vi "WriteLog.vi"(7 "subsystem":string, 8 "data":dbl, 9 "tag":string, 10 "log level":T2(ring)=enum."default", 11 "logger":T1) -> (2 "error code":i32 format="%0.0f", 3 "logger out":T1)   [LabVIEW 2019]
uses:
  Logger.ctl
panel:
  in  "use timestamp? (F)":bool
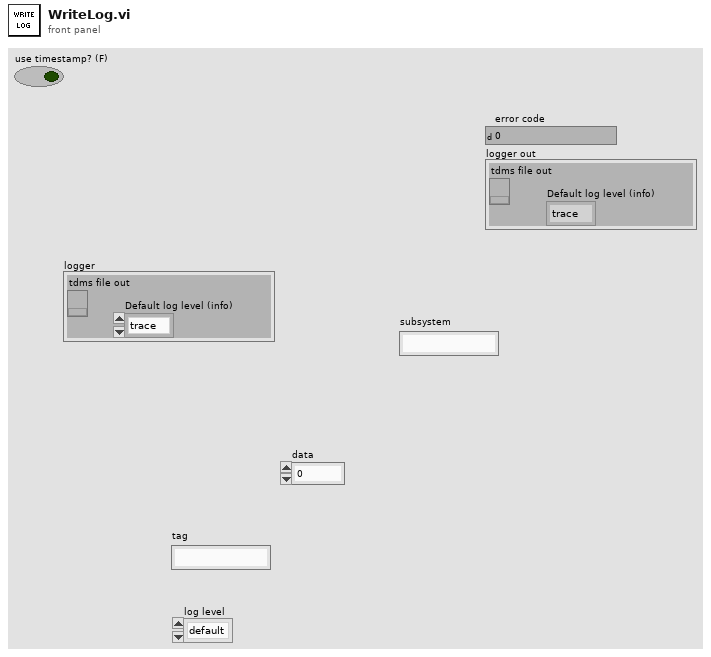
[diagram p1: front panel]
types:
  T1 = typedef "Logger.ctl" = cluster{"tdms file out":refnum<k34>, "Default log level (info)":enum16{"trace", "debug", "info", "warn", "error"}}
  T2 = enum16{"trace", "debug", "info", "warn", "error", "default"}
  T3 = enum16{"trace", "debug", "info", "warn", "error"}
  T4 = enum16{"trace", "debug", "info", "warn", "error", "default"}[]
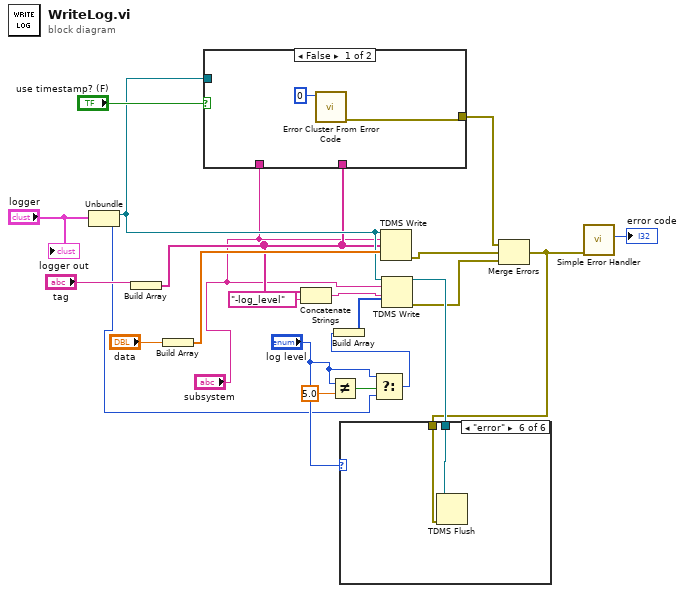
[diagram p0: block diagram]
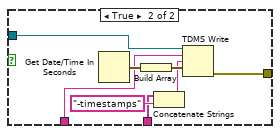
[diagram p7: hidden frame]
diagram:
  n1 = Unbundle("logger") -> ("tdms file out"=w17:refnum<k34>, "Default log level (info)"=w8:T3)
  n2 = Build Array("tag") -> (w16:string[])
  n3 = Build Array("data") -> (w19:dbl[])
  n4 = case shown="False" "use timestamp? (F)" {
    tunnel: w17 -> [_ w30]
    tunnel: w16 -> [_ w28]
    tunnel: "subsystem" -> [_ w26]
    tunnel: [w23 w25] -> w5
    frame False {
      n5 = call <vilib>:"Error Cluster From Error Code.vi"("error code (0)"=0) -> ("error out"=w23:errorcluster)  [unwired: 8 in]
    }
    frame True {
      n6 = Get Date/Time In Seconds() -> (seconds since 1Jan1904=w32:timestamp)
      n7 = Build Array(w32) -> (w31:timestamp[])
      n8 = Concatenate Strings(w28, "-timestamps" ("string")) -> (w27:string)
      n9 = TDMS Write(0:w30, 5:w26, 7:w27, 9:w31) -> (15:w25:errorcluster)  [unwired: 2 in, 3 out]
    }
  }
  n10 = Concatenate Strings(w16, "-log_level" ("string")) -> (w14:string)
  n11 = Not Equal?(x="log level", y=5.0) -> (x != y?=w10:bool)
  n12 = Select(t="log level", s=w10, f=w8) -> (s? t:f=w7:T2)
  n13 = Build Array(w7) -> (w18:T4)
  n14 = TDMS Write(0:w17, 5:"subsystem", 7:w16, 9:w19) -> (15:w4:errorcluster)  [unwired: 2 in, 3 out]
  n15 = TDMS Write(0:w17, 5:"subsystem", 7:w14, 9:w18) -> (4:w12:refnum<k34>, 15:w3:errorcluster)  [unwired: 2 in, 2 out]
  n16 = Merge Errors(w5, w4, w3) -> (w1:errorcluster)
  n17 = case shown="\"error\"" "log level" {
    tunnel: w12 -> [_ _ _ _ _ w34]
    tunnel: w1 -> [_ _ _ _ _ w33]
    frame "default", Default {
    }
    frame "trace" {
    }
    frame "debug" {
    }
    frame "info" {
    }
    frame "warn" {
    }
    frame "error" {
      n18 = TDMS Flush(4:w33, 7:w34) -> ()  [unwired: 2 out]
    }
  }
  n19 = call <vilib>:"Simple Error Handler.vi"("error in (no error)"=w1) -> ("code out"=→"error code":i32)  [unwired: 4 in, 4 out]
  "logger out" <- "logger"
